vi "tmp_toml_exists.vi"(4 "vi":refnum<vi>, 8 "error in (no error)":errorcluster, 11 "path in":path) -> (0 "error out":errorcluster, 1 "text":string, 2 "file exists":bool, 3 "path out":path)   [LabVIEW 2017]
uses:
  <vilib>/Utility/error.llb/Clear Errors.vi
  <vilib>/Utility/file.llb/Application Directory.vi
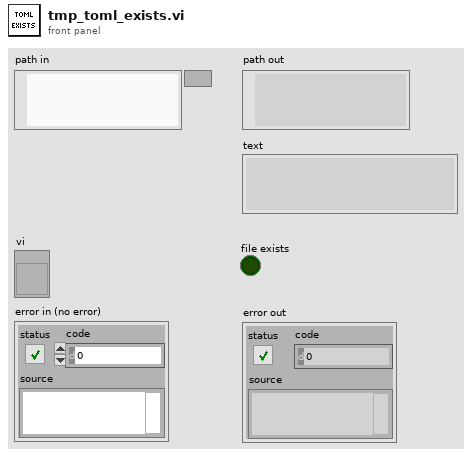
[diagram p1: front panel]
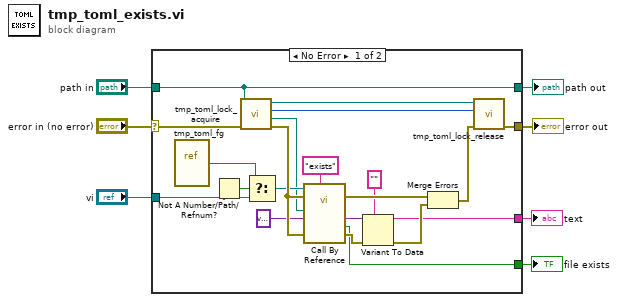
[diagram p0: block diagram]
diagram:
  n1 = case shown="No Error" "error in (no error)" {
    selector: "error in (no error)" -> [w26 w29]
    tunnel: [w22 w29] -> w6
    tunnel: "vi" -> [w19 _]
    tunnel: "path in" -> [w16 w30]
    tunnel: [w16 w30] -> w3
    tunnel: [w13 _] -> w2
    tunnel: [w8 _] -> w1
    frame No Error {
      n2 = vi-ref "tmp_toml_fg.vi"() -> (w18:refnum<vi>)
      n3 = Not A Number/Path/Refnum?(number/path/refnum=w19) -> (NaN/Path/Refnum?=w20:bool)
      n4 = call "tmp_toml_lock_acquire.vi"("error in (no error)"=w26, "path in"=w16) -> ("error out"=w25:errorcluster, "resolved path"=w15:path, "cnt"=w27:u8, "lock"=w28:refnum<queue>)  [unwired: 6 in]
      n5 = Select(t=w18, s=w20, f=w19) -> (s? t:f=w17:refnum<vi>)
      n6 = call-by-ref "?"(reference=w17, error in=w25, "cmd"="exists", 8:"error in (no error)"=w25, "data in"=variant, "path in"=w15) -> (error out=w24:errorcluster, 0:"error out"=w14:errorcluster, "return"=w13:bool, "data out"=w10:variant)  [unwired: 4 in, 2 out]
      n7 = Variant To Data(error in=w14, type="", Variant=w10) -> (data=w8:string, error out=w11:errorcluster)
      n8 = Merge Errors(w24, w11) -> (w23:errorcluster)
      n9 = call "tmp_toml_lock_release.vi"("error in (no error)"=w23, "cnt"=w27, "lock"=w28) -> ("error out"=w22:errorcluster)  [unwired: 8 in]
    }
    frame Error {
    }
  }
  "error out" <- w6
  "path out" <- w3
  "file exists" <- w2
  "text" <- w1
